vi "CheckTest.vi"() -> ()   [LabVIEW 2022 SP3]
uses:
  <userlib>/BS6006PRPLUS_DLL/VIs/Para Pulse.ctl
  <userlib>/BS6006PRPLUS_DLL/VIs/Para TriggerSource.ctl
  <userlib>/BS6006PRPLUS_DLL/BS6006PRPLUS_DLL.lvlib
panel:
  out "TriggerSource":T1
  out "Pulse":T2
  out "Gain (dB)":i32
  out "Trigger delay (£gs)":i32
  out "error out":errorcluster
  out "SamplingFrequency (MHz)":i32
  out "hDevice out":u32
  out "function return":bool
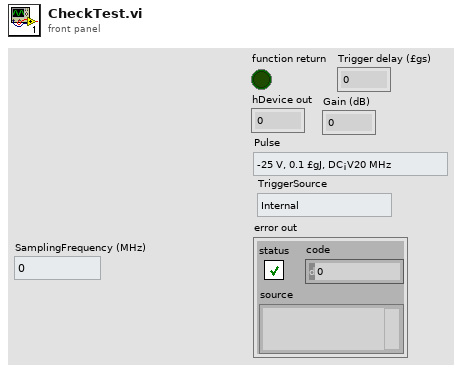
[diagram p1: front panel]
types:
  T1 = typedef "BS6006PRPLUS_DLL.lvlib/Para TriggerSource.ctl" = enum16{"Internal", "External"}
  T2 = typedef "BS6006PRPLUS_DLL.lvlib/Para Pulse.ctl" = enum16{"-25 V, 0.1 £gJ, DC¡V20 MHz", "-45 V, 0.4 £gJ, DC¡V30 MHz", "-75 V, 1.0 £gJ, DC¡V35 MHz", "-120 V, 2.4 £gJ, DC¡V45 MHz", "-190 V, 5.0 £gJ, DC¡V50 MHz", "-190 V, 11 £gJ, DC¡V25 MH", "-190 V, 15 £gJ, DC¡V20 MHz", "-190 V, 20 £gJ, DC¡V15 MHz", "-190 V, 25 £gJ, DC¡V12 MHz", "-190 V, 30 £gJ, DC¡V10 MHz", "-190 V, 40 £gJ, DC¡V8 MHz", "-190 V, 45 £gJ, DC¡V7 MHz", "-190 V, 50 £gJ, DC¡V6 MHz"}
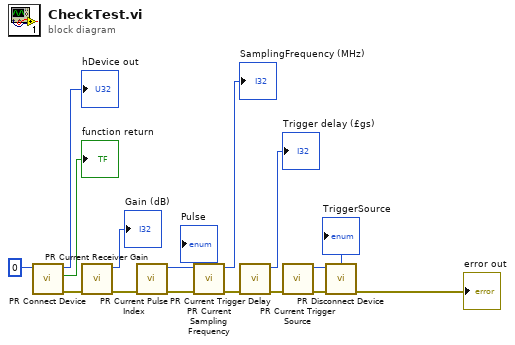
[diagram p0: block diagram]
diagram:
  n1 = call <userlib>:"PR Connect Device.vi"("hDevice"=u32 0) -> ("error out"=w10:errorcluster, "function return"=→"function return":bool, "hDevice out"=→"hDevice out":u32)  [unwired: 8 in]
  n2 = call <userlib>:"PR Current Receiver Gain.vi"("error in (no error)"=w10) -> ("error out"=w15:errorcluster, "Gain (dB)"=→"Gain (dB)":i32)  [unwired: 9 in]
  n3 = call <userlib>:"PR Current Pulse Index.vi"("error in (no error)"=w15) -> ("error out"=w14:errorcluster, "Pulse"=→"Pulse":T2)  [unwired: 9 in]
  n4 = call <userlib>:"PR Current Sampling Frequency.vi"("error in (no error)"=w14) -> ("error out"=w13:errorcluster, "Sampling Frequency (MHz)"=→"SamplingFrequency (MHz)":i32)  [unwired: 9 in]
  n5 = call <userlib>:"PR Current Trigger Delay.vi"("error in (no error)"=w13) -> ("error out"=w12:errorcluster, "Trigger delay (£gs)"=→"Trigger delay (£gs)":i32)  [unwired: 9 in]
  n6 = call <userlib>:"PR Current Trigger Source.vi"("error in (no error)"=w12) -> ("error out"=w11:errorcluster, "TriggerSource"=→"TriggerSource":T1)  [unwired: 9 in]
  n7 = call <userlib>:"PR Disconnect Device.vi"("error in (no error)"=w11) -> ("error out"=→"error out":errorcluster)  [unwired: 10 in]
